vi "tipshaping.action.vi"(8 "Error in (no error)":errorcluster, 11 "TipShapingParam":T1={"TipLift"=-2e-10, "Bias Settling Time"=0.09999999999999999, "Lift Height"=5e-09, "Lift Time 2"=0.2, "Lifting Bias"=2.0, "Lift Time 1"=0.2} {"Lift Time 1" min=0.02 max=600.0 format="%.2p"; "Lifting Bias" format="%.3p"; "Lift Time 2" min=0.02 max=600.0 format="%.2p"; "Lift Height" format="%.2p"; "Bias Settling Time" format="%.2p"; "TipLift" format="%.2p"}) -> (0 "error out":errorcluster, 3 "dz":sgl)   [LabVIEW 2014]
uses:
  <userlib>/Nanonis Prog Interface V5/Nanonis Prog Interface.lvlib
panel:
  out "z channel":i32
  out "initialz":sgl format="%#_6p"
  in  "Feedback":bool=TRUE
  in  "Draw":bool
  in  "Switch Gain":bool
  in  "Current Gain":u16(ring) items=["HS 10^5", "HS 10^6", "HS 10^7", "HS 10^8", "HS 10^9", "HS 10^10", "HS 10^11", "LN 10^3", "LN 10^4", "LN 10^5", "LN 10^6", "LN 10^7", "LN 10^8", "LN 10^9"]
  in  "Bias value":dbl=1.0 format="%.3p"
  in  "Change Bias":bool
  out "Lift Time 1":dbl=0.2 min=0.02 max=600.0 format="%.2p"
  in  "End Wait Time":dbl=0.1 format="%.2p"
  out "Lifting Bias":dbl=2.0 format="%.3p"
  out "Lift Time 2":dbl=0.2 min=0.02 max=600.0 format="%.2p"
  out "Lift Height":dbl=5e-09 format="%.2p"
  out "Bias Settling Time":dbl=0.09999999999999999 format="%.2p"
  out "TipLift":dbl=-2e-10 format="%.2p"
  in  "Switch Off Delay":dbl=0.10999999999999999 format="%.2p"
  out "allQuit":bool
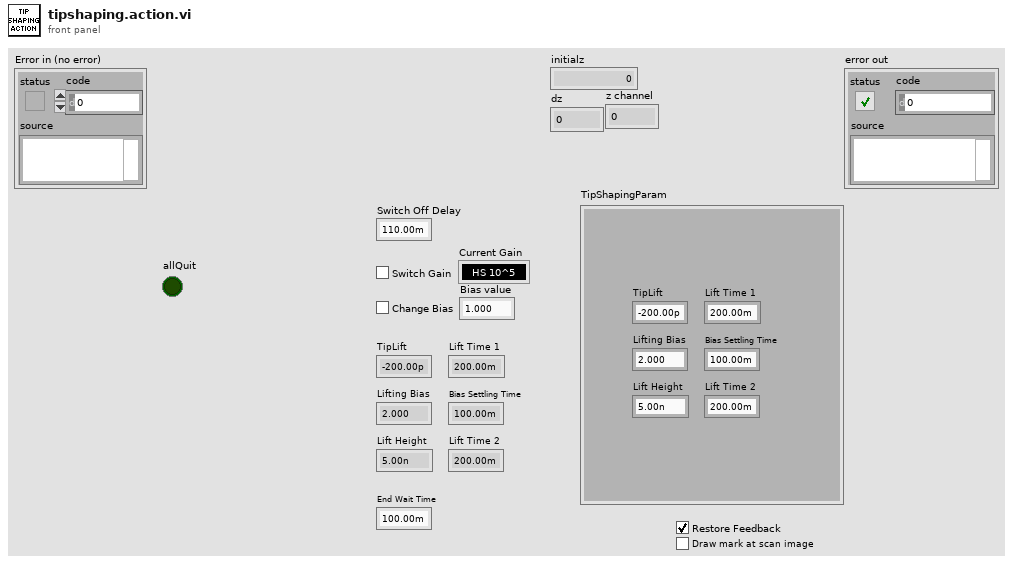
[diagram p1: front panel]
types:
  T1 = cluster{"TipLift":dbl, "Bias Settling Time":dbl, "Lift Height":dbl, "Lift Time 2":dbl, "Lifting Bias":dbl, "Lift Time 1":dbl}
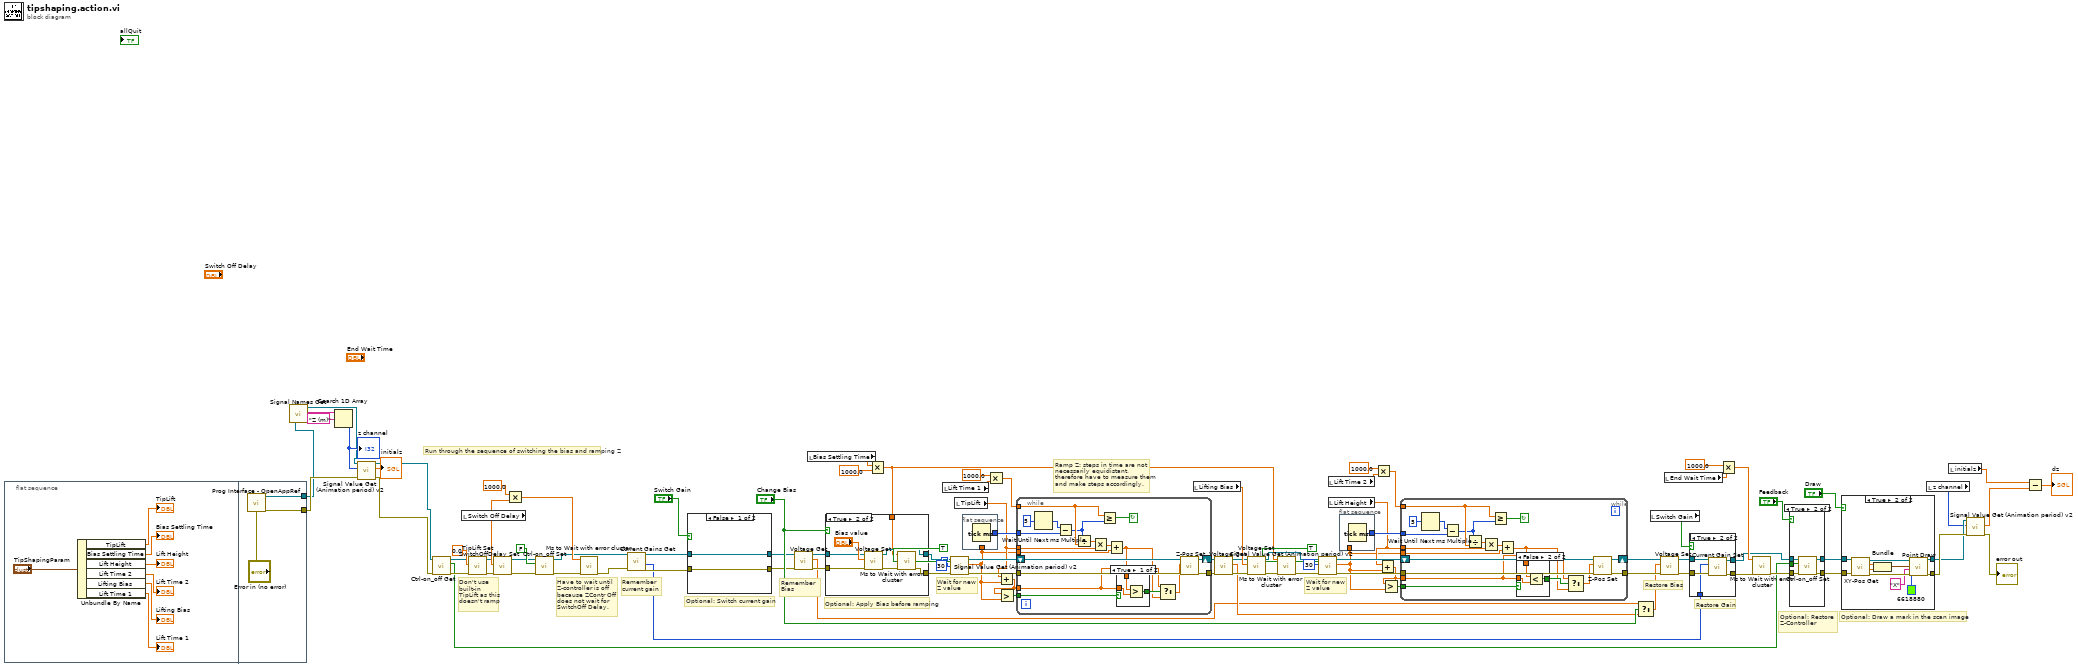
[diagram p0: block diagram]
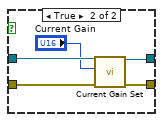
[diagram p4: hidden frame]
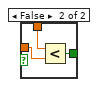
[diagram p6: hidden frame]
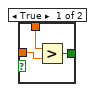
[diagram p8: hidden frame]
diagram:
  # "Ramp Z: steps in time are not necessarily equidistant, therefore have to measure them and make steps accordingly."
  # "Optional: Draw a mark in the scan image"
  # "Optional: Apply Bias before ramping"
  # "Remember Bias"
  # "Optional: Switch current gain"
  # "Remember current gain"
  # "Restore Bias"
  # "Optional: Restore Z-Controller"
  # "Restore Gain"
  # "Don't use built-in TipLift as this doesn't ramp"
  # "Wait for new Z value"
  # "Have to wait until Z-controller is off because ZContr Off does not wait for SwitchOff Delay."
  # "Wait for new Z value"
  # "Run through the sequence of switching the bias and ramping Z"
  n1 = flat-sequence {
    tunnel: [w105] -> w6
    tunnel: [w104] -> w16
    frame #0 {
      n2 = Unbundle By Name("TipShapingParam") -> ("TipLift"=→"TipLift":dbl, "Bias Settling Time"=→"Bias Settling Time":dbl, "Lift Height"=→"Lift Height":dbl, "Lift Time 2"=→"Lift Time 2":dbl, "Lifting Bias"=→"Lifting Bias":dbl, "Lift Time 1"=→"Lift Time 1":dbl)
    }
    frame #1 {
      n3 = call <userlib>:"Prog Interface - OpenAppRef.vi"("Error in (no error)"="Error in (no error)") -> ("Error out"=w104:errorcluster, "Application reference"=w105:refnum<vi>)  [unwired: 5 in]
    }
  }
  n4 = call <userlib>:"Signal Names Get.vi"("Application ref in"=w6) -> ("Signals Names"=w5:string[], "Application ref out"=w2:refnum<vi>)  [unwired: 6 in, 1 out]
  n5 = Search 1D Array(1D array=w5, element="Z (m)") -> (index of element=w3:i32)  [unwired: 1 in]
  "z channel" <- w3
  n6 = call <userlib>:"Signal Value Get (Animation period) v2.vi"("error in (no error)"=w16, "Signal index (0-79)"=w3, "Application ref in"=w2) -> ("error out"=w15:errorcluster, "Signal value"=→"initialz":sgl, "Application ref out"=w14:refnum<vi>)  [unwired: 5 in]
  n7 = call <userlib>:"Ctrl-on_off Get.vi"("error in (no error)"=w15, "Application ref in"=w14) -> ("error out"=w76:errorcluster, "Z-Controller on/off status"=w75:bool, "Application ref out"=w60:refnum<vi>)  [unwired: 7 in]
  n8 = local read "Switch Off Delay"() -> (w84:dbl)
  n9 = call <userlib>:"TipLift Set.vi"("error in (no error)"=w76, "TipLift (m)"=sgl 0.0, "Application ref in"=w60) -> ("error out"=w95:errorcluster, "Application ref out"=w59:refnum<vi>)  [unwired: 7 in]
  n10 = call <userlib>:"SwitchOffDelay Set.vi"("error in (no error)"=w95, "Switch off Delay (s)"=w84, "Application ref in"=w59) -> ("error out"=w66:errorcluster, "Application ref out"=w58:refnum<vi>)  [unwired: 7 in]
  n11 = Multiply(x=1000.0, y=w84) -> (x*y=w74:dbl)
  n12 = call <userlib>:"Ctrl-on_off Set.vi"("error in (no error)"=w66, "Z Controller ON/OFF"=FALSE, "Application ref in"=w58) -> ("error out"=w80:errorcluster, "Application ref out"=w34:refnum<vi>)  [unwired: 7 in]
  n13 = call <userlib>:"Ms to Wait with error cluster.vi"("error in (no error)"=w80, "milliseconds to wait"=w74) -> ("error out"=w32:errorcluster)  [unwired: 4 in, 1 out]
  n14 = call <userlib>:"Current Gains Get.vi"("Error in (no error)"=w32, "Application ref in"=w34) -> ("Error out"=w31:errorcluster, "Selected Gain"=w25:u16, "Application ref out"=w33:refnum<vi>)  [unwired: 6 in, 1 out]
  n15 = case shown="False" "Switch Gain" {
    tunnel: w33 -> [w107 w112]
    tunnel: w31 -> [w106 w111]
    tunnel: [w107 w109] -> w39
    tunnel: [w106 w110] -> w37
    frame False {
    }
    frame True {
      n16 = call <userlib>:"Current Gain Set.vi"("Error in (no error)"=w111, "Gain index"="Current Gain", "Application ref in"=w112) -> ("Error out"=w110:errorcluster, "Application ref out"=w109:refnum<vi>)  [unwired: 7 in]
    }
  }
  n17 = call <userlib>:"Voltage Get.vi"("error in (no error)"=w37, "Application ref in"=w39) -> ("error out"=w36:errorcluster, "Bias (V)"=w35:sgl, "Application ref out"=w38:refnum<vi>)  [unwired: 7 in]
  n18 = local read "Bias Settling Time"() -> (w82:dbl)
  n19 = Multiply(x=w82, y=1000.0) -> (x*y=w43:dbl)
  n20 = case shown="True" "Change Bias" {
    tunnel: w38 -> [w114 w116]
    tunnel: [w114 w120] -> w45
    tunnel: w36 -> [w113 w115]
    tunnel: [w113 w119] -> w44
    tunnel: w43 -> [_ w118]
    frame False {
    }
    frame True {
      n21 = call <userlib>:"Voltage Set.vi"("Error in (no error)"=w115, "Bias (V)"="Bias value", "Application ref in"=w116) -> ("Error out"=w121:errorcluster, "Application ref out"=w120:refnum<vi>)  [unwired: 7 in]
      n22 = call <userlib>:"Ms to Wait with error cluster.vi"("error in (no error)"=w121, "milliseconds to wait"=w118) -> ("error out"=w119:errorcluster)  [unwired: 4 in, 1 out]
    }
  }
  n23 = local read "Lift Time 1"() -> (w64:dbl)
  n24 = call <userlib>:"Signal Value Get (Animation period) v2.vi"("Wait for newest data (F=False)"=TRUE ("Wait for newest data (F)"), "error in (no error)"=w44, "Signal index (0-79)"=i8 30 ("Signal index (0-23)"), "Application ref in"=w45) -> ("error out"=w69:errorcluster, "Signal value"=w22:sgl, "Application ref out"=w56:refnum<vi>)  [unwired: 4 in]
  n25 = local read "TipLift"() -> (w24:dbl)
  n26 = flat-sequence {
    tunnel: [w122] -> w68
    tunnel: w22 -> [_]
    frame #0 {
      n27 = Tick Count (ms)() -> (millisecond timer value=w122:u32)
    }
  }
  n28 = Multiply(x=1000.0, y=w64) -> (x*y=w63:dbl)
  n29 = Add(x=w24, y=w22) -> (x+y=w23:dbl)
  n30 = Greater?(x=w23, y=w22) -> (0:w21:bool)
  n31 = while {
    tunnel: w68 -> [w141]
    tunnel: w24 -> [w139]
    tunnel: [w138] -> w62
    tunnel: w22 -> [w134]
    tunnel: w69 -> [w135]
    tunnel: w63 -> [w132]
    shift-right: [w128] -> w55
    shift-left: w56 -> [w129]
    tunnel: w23 -> [w125]
    tunnel: w21 -> [w127]
    stop <- w140 continue-if-true
    n32 = Wait Until Next ms Multiple(millisecond multiple=u32 5) -> (millisecond timer value=w131:u32)
    n33 = Subtract(x=w131, y=w141) -> (x-y=w130:u32)
    n34 = Divide(x=w130, y=w132) -> (x/y=w136:dbl)
    n35 = Multiply(x=w136, y=w139) -> (x*y=w133:dbl)
    n36 = Greater Or Equal?(x=w132, y=w130) -> (x >= y?=w140:bool)
    n37 = Add(x=w133, y=w134) -> (x+y=w124:dbl)
    n38 = case shown="True" w127 {
      tunnel: w124 -> [w144 w147]
      tunnel: w125 -> [w143 w146]
      tunnel: [w142 w145] -> w126
      frame True {
        n39 = Greater?(x=w144, y=w143) -> (0:w142:bool)
      }
      frame False {
        n40 = Less?(x=w147, y=w146) -> (x < y?=w145:bool)
      }
    }
    n41 = Select(t=w125, s=w126, f=w124) -> (s? t:f=w123:dbl)
    n42 = call <userlib>:"Z-Pos Set.vi"("error in (no error)"=w135, "Z position (m)"=w123, "Application ref in"=w129) -> ("error out"=w138:errorcluster, "Application ref out"=w128:refnum<vi>)  [unwired: 7 in]
  }
  n43 = local read "Lifting Bias"() -> (w94:dbl)
  n44 = call <userlib>:"Voltage Get.vi"("error in (no error)"=w62, "Application ref in"=w55) -> ("error out"=w61:errorcluster, "Bias (V)"=w41:sgl, "Application ref out"=w54:refnum<vi>)  [unwired: 7 in]
  n45 = call <userlib>:"Voltage Set.vi"("Error in (no error)"=w61, "Bias (V)"=w94, "Application ref in"=w54) -> ("Error out"=w79:errorcluster, "Application ref out"=w50:refnum<vi>)  [unwired: 7 in]
  n46 = call <userlib>:"Ms to Wait with error cluster.vi"("error in (no error)"=w79, "milliseconds to wait"=w43) -> ("error out"=w73:errorcluster)  [unwired: 4 in, 1 out]
  n47 = call <userlib>:"Signal Value Get (Animation period) v2.vi"("Wait for newest data (F=False)"=TRUE ("Wait for newest data (F)"), "error in (no error)"=w73, "Signal index (0-79)"=i8 30 ("Signal index (0-23)"), "Application ref in"=w50) -> ("error out"=w72:errorcluster, "Signal value"=w19:sgl, "Application ref out"=w52:refnum<vi>)  [unwired: 4 in]
  n48 = local read "Lift Time 2"() -> (w92:dbl)
  n49 = local read "Lift Height"() -> (w20:dbl)
  n50 = flat-sequence {
    tunnel: [w148] -> w88
    tunnel: w19 -> [_]
    frame #0 {
      n51 = Tick Count (ms)() -> (millisecond timer value=w148:u32)
    }
  }
  n52 = Multiply(x=1000.0, y=w92) -> (x*y=w81:dbl)
  n53 = Add(x=w20, y=w19) -> (x+y=w17:dbl)
  n54 = Greater?(x=w17, y=w19) -> (0:w18:bool)
  n55 = while {
    tunnel: w88 -> [w167]
    tunnel: w20 -> [w165]
    tunnel: [w164] -> w90
    tunnel: w19 -> [w160]
    tunnel: w72 -> [w161]
    tunnel: w81 -> [w158]
    shift-right: [w154] -> w51
    shift-left: w52 -> [w155]
    tunnel: w18 -> [w153]
    tunnel: w17 -> [w150]
    stop <- w166 continue-if-true
    n56 = Wait Until Next ms Multiple(millisecond multiple=u32 5) -> (millisecond timer value=w157:u32)
    n57 = Subtract(x=w157, y=w167) -> (x-y=w156:u32)
    n58 = Divide(x=w156, y=w158) -> (x/y=w162:dbl)
    n59 = Multiply(x=w162, y=w165) -> (x*y=w159:dbl)
    n60 = Greater Or Equal?(x=w158, y=w156) -> (x >= y?=w166:bool)
    n61 = Add(x=w159, y=w160) -> (x+y=w151:dbl)
    n62 = case shown="False" w153 {
      tunnel: w151 -> [w170 w173]
      tunnel: w150 -> [w169 w172]
      tunnel: [w168 w171] -> w152
      frame True {
        n63 = Greater?(x=w170, y=w169) -> (0:w168:bool)
      }
      frame False {
        n64 = Less?(x=w173, y=w172) -> (x < y?=w171:bool)
      }
    }
    n65 = Select(t=w150, s=w152, f=w151) -> (s? t:f=w149:dbl)
    n66 = call <userlib>:"Z-Pos Set.vi"("error in (no error)"=w161, "Z position (m)"=w149, "Application ref in"=w155) -> ("error out"=w164:errorcluster, "Application ref out"=w154:refnum<vi>)  [unwired: 7 in]
  }
  n67 = Select(t=w35, s="Change Bias", f=w41) -> (s? t:f=w40:sgl)
  n68 = local read "Switch Gain"() -> (w30:bool)
  n69 = call <userlib>:"Voltage Set.vi"("Error in (no error)"=w90, "Bias (V)"=w40, "Application ref in"=w51) -> ("Error out"=w27:errorcluster, "Application ref out"=w29:refnum<vi>)  [unwired: 7 in]
  n70 = local read "End Wait Time"() -> (w86:dbl)
  n71 = case shown="True" w30 {
    tunnel: w29 -> [w175 w180]
    tunnel: [w175 w179] -> w28
    tunnel: w27 -> [w174 w178]
    tunnel: [w174 w177] -> w26
    tunnel: w25 -> [_ w176]
    frame False {
    }
    frame True {
      n72 = call <userlib>:"Current Gain Set.vi"("Error in (no error)"=w178, "Gain index"=w176, "Application ref in"=w180) -> ("Error out"=w177:errorcluster, "Application ref out"=w179:refnum<vi>)  [unwired: 7 in]
    }
  }
  n73 = Multiply(x=1000.0, y=w86) -> (x*y=w77:dbl)
  n74 = call <userlib>:"Ms to Wait with error cluster.vi"("error in (no error)"=w26, "milliseconds to wait"=w77) -> ("error out"=w78:errorcluster)  [unwired: 4 in, 1 out]
  n75 = case shown="True" "Feedback" {
    tunnel: w78 -> [w181 w187]
    tunnel: w75 -> [_ w186]
    tunnel: w28 -> [w182 w185]
    tunnel: [w182 w184] -> w48
    tunnel: [w181 w183] -> w47
    frame False {
    }
    frame True {
      n76 = call <userlib>:"Ctrl-on_off Set.vi"("error in (no error)"=w187, "Z Controller ON/OFF"=w186, "Application ref in"=w185) -> ("error out"=w183:errorcluster, "Application ref out"=w184:refnum<vi>)  [unwired: 7 in]
    }
  }
  n77 = case shown="True" "Draw" {
    tunnel: w48 -> [w188 w199]
    tunnel: w47 -> [_ w197]
    tunnel: [w188 w195] -> w11
    tunnel: [_ w189] -> w13
    frame False {
    }
    frame True {
      n78 = call <userlib>:"XY-Pos Get.vi"("error in (no error)"=w197, "Application ref in"=w199) -> ("error out"=w196:errorcluster, "Y (m)"=w193:sgl, "X (m)"=w194:sgl, "Application ref out"=w198:refnum<vi>)  [unwired: 5 in]
      n79 = Bundle("X (m)"=w194, "Y (m)"=w193) -> (w192:cluster{"X (m)":sgl, "Y (m)":sgl})  [unwired: 1 in]
      n80 = call <userlib>:"Point Draw.vi"("Application ref in"=w198, "Point Coordinates"=w192, "Text"="X", "Color"=u32 6618880, "error in (no error)"=w196) -> ("Application ref out"=w195:refnum<vi>, "error out"=w189:errorcluster)  [unwired: 9 in]
    }
  }
  n81 = local read "z channel"() -> (w1:i32)
  n82 = local read "initialz"() -> (w9:sgl)
  n83 = call <userlib>:"Signal Value Get (Animation period) v2.vi"("error in (no error)"=w13, "Signal index (0-79)"=w1, "Application ref in"=w11) -> ("error out"=→"error out":errorcluster, "Signal value"=w8:sgl)  [unwired: 5 in, 1 out]
  n84 = Subtract(x=w9, y=w8) -> (x-y=→"dz":sgl)
